vi "Abstract MVA Application Template.vi"() -> ()   [LabVIEW 2019]
uses:
  <vilib>/gpm_packages/@cs/mva-core/Source/IModel/IModel/IModel.lvclass
  C:/Program Files/National Instruments/LabVIEW 2019/vi.lib/gpm_packages/@cs/mva-core/Source/IObserver/IObserver/IObserver.lvclass
  <vilib>/gpm_packages/@cs/mva-viewable/Source/IViewable/IViewable/IViewable.lvclass
  <vilib>/gpm_packages/@cs/mva-viewable/Source/IViewModel/IViewModel/IViewModel.lvclass
  C:/Program Files/National Instruments/LabVIEW 2019/vi.lib/gpm_packages/@cs/mva-viewable/Source/IViewManager/IViewManager/IViewManager.lvclass
  C:/Program Files/National Instruments/LabVIEW 2019/vi.lib/ActorFramework/Actor/Actor.lvclass
  <vilib>/gpm_packages/@cs/mva-core/Source/MonitoredMediator/MonitoredMediator/MonitoredMediator.lvclass
  C:/Program Files/National Instruments/LabVIEW 2019/vi.lib/gpm_packages/@cs/mva-core/Source/IMediator/IMediator/IMediator.lvclass
  <vilib>/ActorFramework/Message Enqueuer/Message Priority.ctl
  <vilib>/gpm_packages/@cs/mva-viewable/Source/IViewable/IViewable/View Position Enum.ctl
  <vilib>/gpm_packages/@cs/BusMonitor/ListboxBusMonitor/ListboxBusMonitor/ListboxBusMonitor.lvclass/ListboxBusMonitor.ctl
  <vilib>/gpm_packages/@cs/event-logger/Source/ConsoleView/View/TypeDef/String Config.ctl
  <vilib>/gpm_packages/@cs/event-logger/Source/Composed Log/Types/Log Level.ctl
  <vilib>/gpm_packages/@cs/event-logger/Source/Composed Log/Log Sink/Sink Error Actions ENUM.ctl
  <vilib>/gpm_packages/@cs/event-logger/Source/Text File Sink/Configuration.ctl
  <vilib>/gpm_packages/@cs/mva-core/Source/MonitoredMediator/MonitoredMediator/MonitoredMediator.lvclass/MonitoredMediator.ctl
  <vilib>/gpm_packages/@cs/event-logger/Source/Composed Log/LoggerReference/LoggerReference.lvclass/LoggerReference.ctl
  <vilib>/gpm_packages/@cs/mva-core/Source/IObserver/IObserver/IObserver.lvclass/IObserver.ctl
  <vilib>/gpm_packages/@cs/mva-core/Source/IMediator/IMediator/IMediator.lvclass/IMediator.ctl
  <vilib>/gpm_packages/@cs/mva-viewable/Source/IViewModel/IViewModel/IViewModel.lvclass/IViewModel.ctl
  <vilib>/gpm_packages/@cs/mva-viewable/Source/IViewManager/IViewManager Messages/Launch Nested Views Msg/Launch Nested Views Msg.lvclass/Launch Nested Views Msg.ctl
  <vilib>/gpm_packages/@cs/mva-viewable/Source/IViewManager/IViewManager/IViewManager.lvclass/IViewManager.ctl
  <vilib>/gpm_packages/@cs/mva-viewable/Source/IViewable/IViewable Messages/Open Front Panel Msg/Open Front Panel Msg.lvclass/Open Front Panel Msg.ctl
  <vilib>/ActorFramework/Message Enqueuer/Message Enqueuer.lvclass/Message Enqueuer.ctl
  8aeb1c73-ee09-4c42-9ba4-2ac02e328119.vi
  5c4f144a-bf04-4631-b5b9-56dc2cdea438.vi
  <vilib>/gpm_packages/@cs/mva-core/Source/MonitoredMediator/MonitoredMediator/Private Write BusMonitors.vi
  5c4f144a-bf04-4631-b5b9-56dc2cdea438.vi/0be720b3-07b8-4c20-b2f5-faff34d5f1a2.vi
  <vilib>/gpm_packages/@cs/mva-core/Source/IObserver/IObserver/Configure Observer Logging.vi
  <vilib>/gpm_packages/@cs/mva-viewable/Source/IViewModel/IViewModel/Write Startup Model-View Configuration.vi
  <vilib>/gpm_packages/@cs/mva-core/Source/IMediator/IMediator/Configure Mediator.vi
  <vilib>/ActorFramework/Message Enqueuer/Enqueue.vi
  <vilib>/gpm_packages/@cs/event-logger/Source/Composed Log/LoggerReference/Return Aggregate Queues.vi
  <vilib>/gpm_packages/@cs/event-logger/Source/Composed Log/LoggerReference/Add Aggregate Log.vi
  5c4f144a-bf04-4631-b5b9-56dc2cdea438.vi/0be720b3-07b8-4c20-b2f5-faff34d5f1a2.vi/b8b1fb38-4ada-4e37-8009-dc8e5027a422.vi
  <vilib>/gpm_packages/@cs/mva-viewable/Source/IViewManager/IViewManager Messages/Launch Nested Views Msg/Pack Launch Nested Views Msg.vi
  <vilib>/gpm_packages/@cs/mva-viewable/Source/IViewManager/IViewManager/Write Startup Launch Nested Views Msg.vi
  <vilib>/gpm_packages/@cs/event-logger/Source/Composed Log/LoggerReference/Send Add Sink.vi
  <vilib>/gpm_packages/@cs/event-logger/Source/Text File Sink/Text File Sink.lvclass
  C:/Program Files/National Instruments/LabVIEW 2019/vi.lib/gpm_packages/@cs/event-logger/Source/Composed Log/Log Sink/Log Sink.lvclass
  <vilib>/gpm_packages/@cs/event-logger/Source/ConsoleView/Sink/ConsoleSink.lvclass
  <vilib>/gpm_packages/@cs/mva-viewable/Source/IViewable/IViewable Messages/Open Front Panel Msg/Open Front Panel Msg.lvclass
  C:/Program Files/National Instruments/LabVIEW 2019/vi.lib/ActorFramework/Message/Message.lvclass
  <vilib>/gpm_packages/@cs/event-logger/Source/Composed Log/Application Logger/Launch Worker Loop.vi
  <vilib>/gpm_packages/@cs/event-logger/Source/Composed Log/LoggerReference/Initialize Logger Instance.vi
  <vilib>/ActorFramework/Message Priority Queue/Priority Enqueue.vi
  <vilib>/gpm_packages/@cs/BusMonitor/ListboxBusMonitor/ListboxBusMonitor/ListboxBusMonitor.lvclass
  <vilib>/gpm_packages/@cs/event-logger/Source/Composed Log/LoggerReference/LoggerReference.lvclass
  <vilib>/gpm_packages/@cs/event-logger/Source/Composed Log/IErrorFormat/IErrorFormat.lvclass
  <vilib>/gpm_packages/@cs/event-logger/Source/Composed Log/Log Sink/Log Sink.lvclass
  <vilib>/gpm_packages/@cs/mva-viewable/Source/IViewable/IApplicationStyle/IApplicationStyle.lvclass
  <vilib>/gpm_packages/@cs/mva-viewable/Source/IViewManager/IViewManager Messages/Launch Nested Views Msg/Launch Nested Views Msg.lvclass
  <vilib>/ActorFramework/Actor/Actor.lvclass
  <vilib>/ActorFramework/Message Enqueuer/Message Enqueuer.lvclass
  <vilib>/gpm_packages/@cs/event-logger/Source/ConsoleView/ConsoleInterface/ConsoleSession.lvclass
  <vilib>/gpm_packages/@cs/event-logger/Source/ConsoleView/View/ConsoleView.lvclass
  <vilib>/gpm_packages/@cs/event-logger/Source/Composed Log/Composed Log.lvlib
panel:
  out "Application:Directory Path":path
  # "This example launches a simple abstract MVA application.\nReplace IModel with your Root Model or dependency-injected Model hierarchy.\nReplace IViewable with your Viewable or nested hierarchy of Viewables and ViewManagers\nReplace IViewModel with your concrete ViewModel that requests Model activity driven by user inputs\nMediator is already concrete--only replace it if you write your own Mediator"
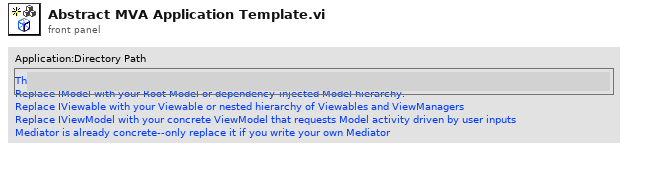
[diagram p1: front panel]
types:
  T1 = typedef "Text File Sink.lvclass/Configuration.ctl" = cluster{"Folder":path, "Name":string, "Extension":string, "Max Size (MB)":i64, "Timestamp Filename":bool}
  T2 = typedef "Composed Log.lvlib/Log Sink.lvclass/Sink Error Actions ENUM.ctl" = enum16{"Ignore Error and Continue", "Ignore Error and Close Sink", "Report Error and Close Sink"}
  T3 = typedef "Composed Log.lvlib/Log Level.ctl" = enum16{"Debug", "Info", "Warning", "Error", "Critical"}
  T4 = typedef "ConsoleView.lvlib/ConsoleView.lvclass/String Config.ctl" = cluster{"BG Color":u32, "Text Color":u32, "Font Size":u32, "Bold?":bool}
  T5 = typedef "IViewable.lvlib/IViewable.lvclass/View Position Enum.ctl" = enum16{"Centered", "Maximized", "Minimized", "Custom", "Unchanged"}
  T6 = typedef "Actor Framework.lvlib/Message Enqueuer.lvclass/Message Priority.ctl" = enum16{"Low", "Normal", "High"}
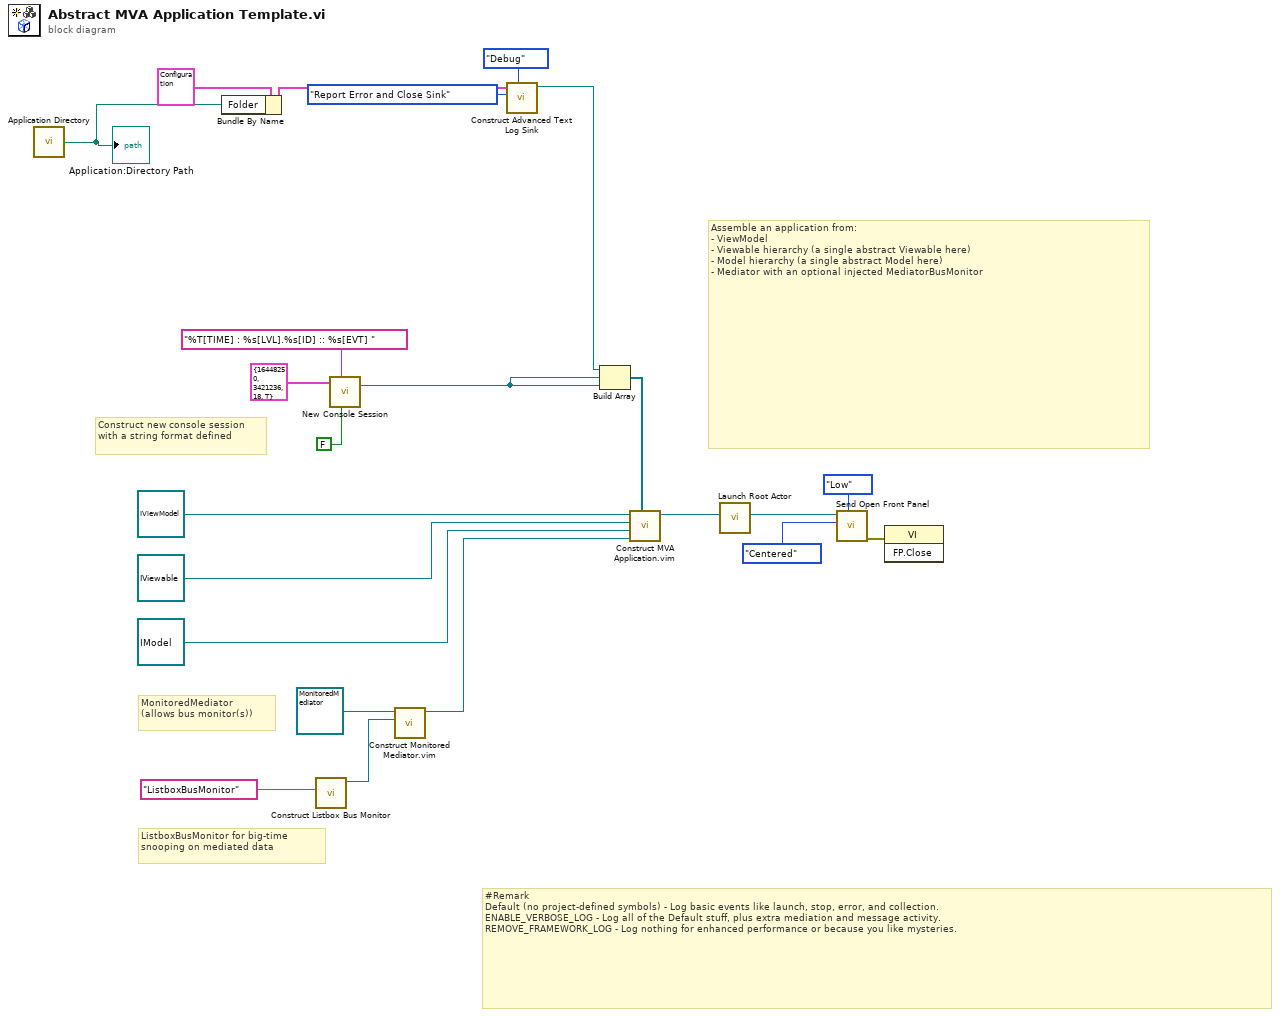
[diagram p0: block diagram]
diagram:
  # "Construct new console session with a string format defined"
  # "ListboxBusMonitor for big-time\nsnooping on mediated data"
  # "MonitoredMediator\n(allows bus monitor(s))"
  # "#Remark \nDefault (no project-defined symbols) - Log basic events like launch, stop, error, and collection.\nENABLE_VERBOSE_LOG - Log all of the Default stuff, plus extra mediation and message activity.\nREMOVE_FRAMEWORK_LOG - Log nothing for enhanced performance or because you like mysteries."
  # "Assemble an application from:\n- ViewModel\n- Viewable hierarchy (a single abstract Viewable here)\n- Model hierarchy (a single abstract Model here)\n- Mediator with an optional injected MediatorBusMonitor"
  n1 = call <vilib>:"Application Directory.vi"() -> ("Application Directory"=w2:path)
  "Application:Directory Path" <- w2
  n2 = Bundle By Name(cluster=T1 {"Folder"=path "", "Name"="Event Log", "Extension"="txt", "Max Size (MB)"=1, "Timestamp Filename"=TRUE} ("Text File Configuration"), "Folder"=w2) -> (w3:T1)
  n3 = call <vilib>:"Construct Listbox Bus Monitor.vi"("Show Panel Boolean Name"="ListboxBusMonitor") -> ("ListboxBusMonitor out"=w14:refnum<class "ListboxBusMonitor.lvclass">)  [unwired: 10 in]
  n4 = call <vilib>:"New Console Session.vi"("Persist After Shutdown?(F)"=FALSE, "Format Specifier"="%T[TIME] : %s[LVL].%s[ID] :: %s[EVT] ", "UI Config"=T4 {"BG Color"=16448250, "Text Color"=3421236, "Font Size"=18, "Bold?"=TRUE}) -> ("ConsoleSink out"=w1:refnum<class "ConsoleSink.lvclass">)  [unwired: 6 in, 2 out]
  n5 = call "Construct Monitored Mediator.vim"("Startup Bus Monitor(s)"=w14, "MonitoredMediator in"=refnum<class "MonitoredMediator.lvclass"> refnum ("MonitoredMediator.lvlib:MonitoredMediator.lvclass")) -> ("MonitoredMediator out"=w15:refnum<class "MonitoredMediator.lvclass">)  [unwired: 9 in]
  n6 = call <vilib>:"Construct Advanced Text Log Sink.vi"("LogLevel"=Log_Level."Debug", "Error Action"=Sink_Error_Actions_ENUM."Report Error and Close Sink", "Text File Configuration"=w3) -> ("Text File Sink out"=w7:refnum<class "Text File Sink.lvclass">)  [unwired: 8 in]
  n7 = Build Array(w7, w1, w1) -> (w8:refnum<class "Log Sink.lvclass">[])
  n8 = call "Construct MVA Application.vim"("Event Log Sink(s)"=w8, "Mediator Type"=w15, "Model Type"=refnum<class "IModel.lvclass"> refnum ("IModel.lvlib:IModel.lvclass"), "Startup View Configuration"=refnum<class "IViewable.lvclass"> refnum ("IViewable.lvlib:IViewable.lvclass"), "IViewModel In"=refnum<class "IViewModel.lvclass"> refnum ("IViewModel.lvlib:IViewModel.lvclass")) -> ("IViewModel Out"=w20:refnum<class "IViewModel.lvclass">)  [unwired: 6 in]
  n9 = call <vilib>:"Launch Root Actor.vi"("Actor"=w20) -> ("Actor's Enqueuer"=w19:refnum<class "Message Enqueuer.lvclass">)  [unwired: 9 in, 1 out]
  n10 = call <vilib>:"Send Open Front Panel.vi"("Message Priority (Normal)"=Message_Priority."Low", "Position"=View_Position_Enum."Centered", "Message Enqueuer"=w19) -> ("error out"=w9:errorcluster)  [unwired: 7 in, 1 out]
  n11 = invoke class="VI" method="FP.Close"(error in=w9) -> ()  [unwired: 2 in, 3 out]
